vi "Write 7z config.vi"(8 "error in (no error)":errorcluster, 11 "PostBuildSupport in":refnum<class "PostBuildSupport.lvclass">) -> (0 "error out":errorcluster, 3 "PostBuildSupport out":refnum<class "PostBuildSupport.lvclass">)   [LabVIEW 2016, in "build support.lvlib" / "PostBuildSupport.lvclass"]
uses:
  PostBuildSupport.lvclass
  PostBuildSupport.lvclass/PostBuildSupport.ctl
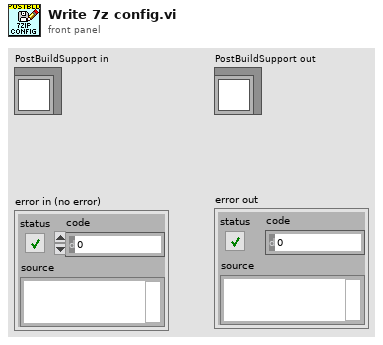
[diagram p1: front panel]
types:
  T1 = enum16{"open", "replace", "create", "open or create", "replace or create", "replace or create with confirmation"}
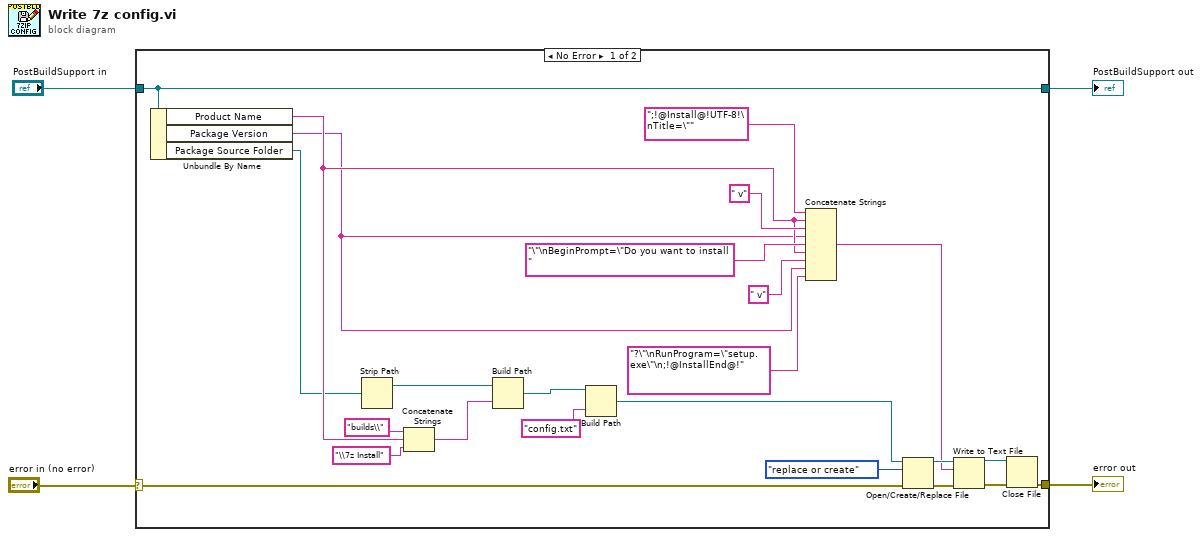
[diagram p0: block diagram]
diagram:
  n1 = case shown="No Error" "error in (no error)" {
    selector: "error in (no error)" -> [w5 w29]
    tunnel: [w18 w29] -> w4
    tunnel: "PostBuildSupport in" -> [w6 w30]
    tunnel: [w6 w30] -> w2
    frame No Error {
      n2 = Unbundle By Name(w6) -> ("Product Name"=w9:string, "Package Version"=w7:string, "Package Source Folder"=w8:path)
      n3 = Strip Path(path=w8) -> (stripped path=w27:path)  [unwired: 1 out]
      n4 = Concatenate Strings("builds\\" ("name or relative path"), w9, "\\7z Install" ("name or relative path")) -> (w10:string)
      n5 = Build Path(base path=w27, name or relative path=w10) -> (appended path=w17:path)
      n6 = Build Path(base path=w17, name or relative path="config.txt") -> (appended path=w22:path)
      n7 = Concatenate Strings(";!@Install@!UTF-8!\nTitle=\"" ("Name of target (My Computer)"), w9, " v" ("Name of target (My Computer)"), w7, "\"\nBeginPrompt=\"Do you want to install " ("Name of target (My Computer)"), w9, " v" ("Name of target (My Computer)"), w7, "?\"\nRunProgram=\"setup.exe\"\n;!@InstallEnd@!" ("Name of target (My Computer)")) -> (w24:string)
      n8 = Open/Create/Replace File(file path (use dialog)=w22, error in=w5, operation (0:open)=T1."replace or create") -> (refnum out=w25:refnum<file>, error out=w23:errorcluster)  [unwired: 3 in, 1 out]
      n9 = Write to Text File(file (use dialog)=w25, text=w24, error in=w23) -> (refnum out=w19:refnum<file>, error out=w20:errorcluster)  [unwired: 1 in, 1 out]
      n10 = Close File(refnum=w19, error in=w20) -> (error out=w18:errorcluster)  [unwired: 1 out]
    }
    frame Error {
    }
  }
  "error out" <- w4
  "PostBuildSupport out" <- w2
